vi "3 Matrix RGB.vi"() -> ()   [LabVIEW 2019]
uses:
  <vilib>/FPGAPlugInAG/myRIO-1900/niLvFpga_Open_myRIO-1900.vi
  <vilib>/rvi/interface/common/dynamic/niFpgaDynamicAddResources.vi
  <vilib>/Utility/error.llb/Error Cluster From Error Code.vi
  <vilib>/rvi/errors/niLvFpgaAdjustHostInterfaceError.vi
  <vilib>/FPGAPlugInAG/Dynamic/niLvFpga_Close_Dynamic.vi
  <vilib>/rvi/interface/nirviOpenFPGA/nirviOpenFPGA.xnode
  FPGA Bitfiles/myrio-neopixel_FPGATarget_TestNeopixel_-8uHP6HNTAw.lvbitx
  <vilib>/rvi/interface/nirviReadWriteControl/nirviReadWriteControl.xnode
  <vilib>/rvi/interface/nirviMethod/nirviMethod.xnode
  <vilib>/rvi/interface/nirviCloseFPGA/nirviCloseFPGA.xnode
  LED Matrix Host/LED Matrix Host.lvlib
  <vilib>/FPGAPlugInAG/Dynamic/niLvFpga_WriteFifo_Dynamic.vi
  <vilib>/rvi/errors/niLvFpgaMergeErrorWithErrorCode.vi
  NiFpgaLv.dll
  <vilib>/rvi/interface/Simulation/niFpgaSimulationCallBeginRW.vi
panel:
  in  "Color Box":u32(colorbox)=6618880
  in  "FPS":u32(slide)=8 scale=0.0..100.0
  in  "Update":bool=TRUE
  in  "stop":bool
  in  "Intensity":sgl(slide)=0.20433436 scale=0.0..1.0
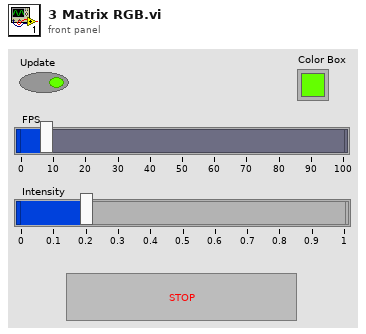
[diagram p1: front panel]
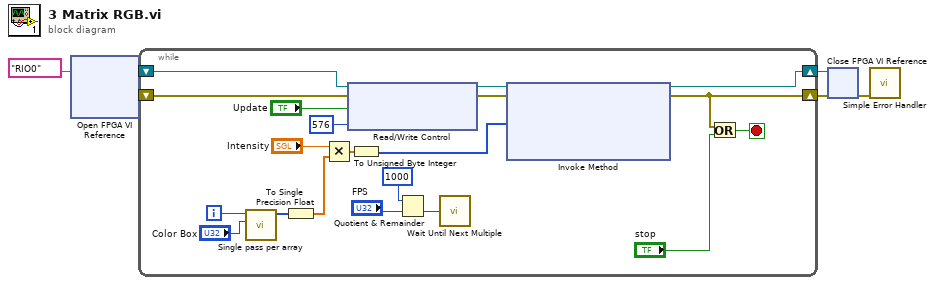
[diagram p0: block diagram]
diagram:
  n1 = xnode "Open FPGA VI Reference"("resource name"=tag "RIO0") -> ("FPGA VI Reference Out"=w2:refnum<k20>, "error out"=w1:errorcluster)  [unwired: 1 in]
  n2 = while {
    shift-right: [w14] -> w6
    shift-left: w2 -> [w26]
    shift-right: [w9] -> w5
    shift-left: w1 -> [w25]
    i -> [w12]
    stop <- w7 stop-if-true
    n3 = call "Single pass per array.vi"("Color Box"="Color Box", "index"=w12) -> ("Raw Data"=w11:u8[])  [unwired: 9 in]
    n4 = To Single Precision Float(number=w11) -> (single precision float=w21:sgl[])
    n5 = Multiply(x="Intensity", y=w21) -> (x*y=w22:sgl[])
    n6 = xnode "Read/Write Control"("FPGA VI Reference In"=w26, "error in"=w25, "Update"="Update", "Number Of Elements"=576) -> ("FPGA VI Reference Out"=w16:refnum<k20>, "error out"=w15:errorcluster)
    n7 = To Unsigned Byte Integer(number=w22) -> (unsigned 8bit integer=w10:u8[])
    n8 = Quotient & Remainder(x=u32 1000 ("y"), y="FPS") -> (floor(x/y)=w18:u32)  [unwired: 1 out]
    n9 = call "Wait Until Next Multiple"("Count(mSec)"=w18) -> ()  [unwired: 1 out]
    n10 = xnode "Invoke Method"("FPGA VI Reference In"=w16, "error in"=w15, "Data"=w10) -> ("FPGA VI Reference Out"=w14:refnum<k20>, "error out"=w9:errorcluster)  [unwired: 1 in, 1 out]
    n11 = Or(x=w9, y="stop") -> (x .or. y?=w7:bool)
  }
  n12 = xnode "Close FPGA VI Reference"("FPGA VI Reference In"=w6, "error in"=w5) -> ("error out"=w4:errorcluster)
  n13 = call <vilib>:"Simple Error Handler.vi"("error in (no error)"=w4) -> ()  [unwired: 4 in, 5 out]
